vi "Section99_EXIT-01_CloseReferences.vi"(8 "error in (no error)":errorcluster, 11 "ShiftRegister in":T1) -> (0 "error out":errorcluster)   [LabVIEW 2014, in "GUIUpdateQSM.lvlib"]
uses:
  GUIUpdateQSM.lvlib
  Controls/QSM_ShiftRegister.ctl
  QueueMaintenance/TypeDef/QSMRef_ALL.ctl
  Controls/QSM_Reference.ctl
  Controls/QSM_DataType.ctl
  Controls/QSM_RunStates.ctl
  Queue_TEST/Controls/QSM_Reference.ctl
  Queue_TEST/Controls/QSM_DataType.ctl
  Queue_TEST/Controls/QSM_RunStates.ctl
  Controls/TypeDef_FrontPanelReferences.ctl
  Queue_TEST/TestQSM.lvlib
  QueueMaintenance/QueueMaintenance.lvlib
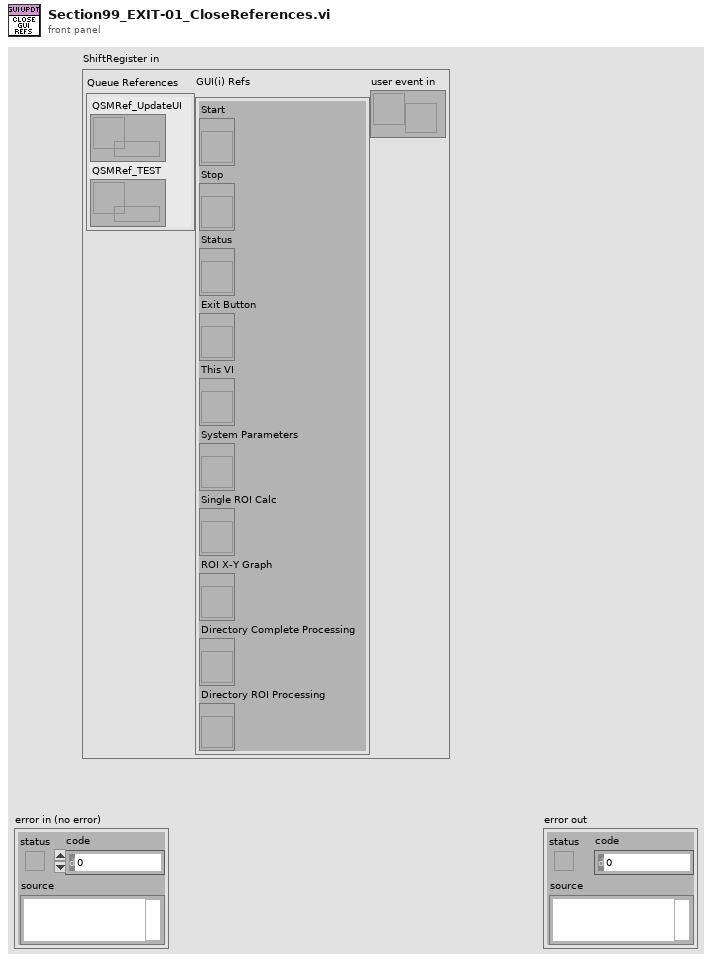
[diagram p1: front panel]
types:
  T1 = typedef "GUIUpdateQSM.lvlib/QSM_ShiftRegister.ctl" = cluster{"Queue References":T2, "GUI(i) Refs":T5, "user event in":refnum<user-event>}
  T2 = typedef "QueueMaintenance.lvlib/QSMRef_ALL.ctl" = cluster{"QSMRef_UpdateUI":T3, "QSMRef_TEST":T4}
  T3 = typedef "GUIUpdateQSM.lvlib/QSM_Reference.ctl" = refnum<queue>
  T4 = typedef "TestQSM.lvlib/QSM_Reference.ctl" = refnum<queue>
  T5 = typedef "GUIUpdateQSM.lvlib/TypeDef_FrontPanelReferences.ctl" = cluster{"Start":refnum<vi>, "Stop":refnum<vi>, "Status":refnum<vi>, "Exit Button":refnum<vi>, "This VI":refnum<vi>, "System Parameters":refnum<vi>, "Single ROI Calc":refnum<vi>, "ROI X-Y Graph":refnum<vi>, "Directory Complete Processing":refnum<vi>, "Directory ROI Processing":refnum<vi>}
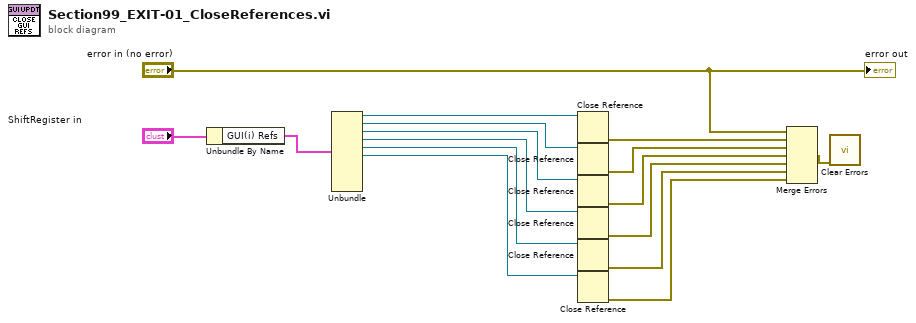
[diagram p0: block diagram]
diagram:
  n1 = Unbundle By Name("ShiftRegister in") -> ("GUI(i) Refs"=w3:T5)
  n2 = Unbundle(w3) -> ("Start"=w10:refnum<vi>, "Stop"=w9:refnum<vi>, "Status"=w8:refnum<vi>, "Exit Button"=w7:refnum<vi>, "This VI"=w6:refnum<vi>, "System Parameters"=w5:refnum<vi>)  [unwired: 4 out]
  n3 = Close Reference(reference=w10) -> (error out=w16:errorcluster)  [unwired: 1 in]
  n4 = Close Reference(reference=w9) -> (error out=w15:errorcluster)  [unwired: 1 in]
  n5 = Close Reference(reference=w8) -> (error out=w14:errorcluster)  [unwired: 1 in]
  n6 = Close Reference(reference=w7) -> (error out=w13:errorcluster)  [unwired: 1 in]
  n7 = Close Reference(reference=w6) -> (error out=w12:errorcluster)  [unwired: 1 in]
  n8 = Close Reference(reference=w5) -> (error out=w11:errorcluster)  [unwired: 1 in]
  n9 = Merge Errors("error in (no error)", w16, w15, w14, w13, w12, w11) -> (w1:errorcluster)
  n10 = call <vilib>:"Clear Errors.vi"("error in (no error)"=w1) -> ()  [unwired: 5 in, 2 out]
  "error out" <- "error in (no error)"
